vi "StateLimeLight.vi"(0 "Master State":enum16{"Normal", "Climb"}(ring)) -> ()   [LabVIEW 2020]
doc: "This VI manages the LimeLight pipelines and LimeLight targeting LED mode."
uses:
  driverdata.vi
  sensordata.vi
  robotoutputs.vi
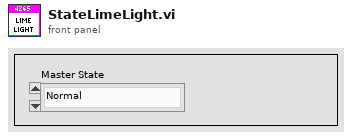
[diagram p1: front panel]
types:
  T1 = enum16{"Robot-Oriented", "Field-Oriented", "Intake"}
  T2 = enum16{"Side-by-Side", "PiP Main", "PiP Secondary"}
  T3 = enum16{"Boot Up", "Camera Override", "HUB Targeting", "CARGO Tracking"}
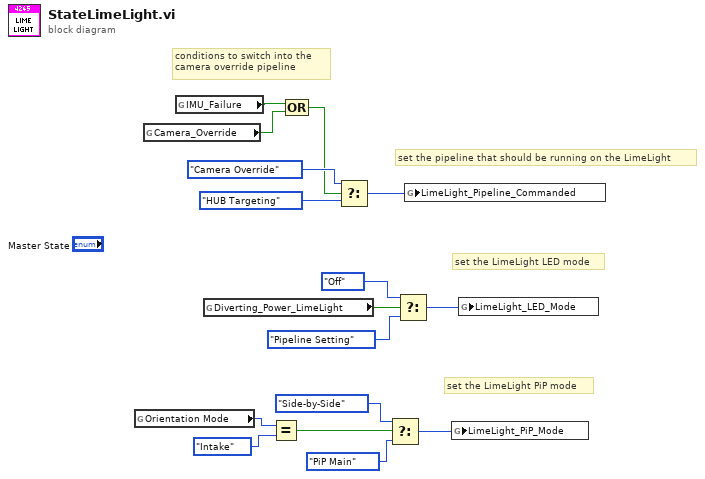
[diagram p0: block diagram]
diagram:
  # "set the LimeLight PiP mode"
  # "set the LimeLight LED mode"
  # "conditions to switch into the \ncamera override pipeline"
  # "set the pipeline that should be running on the LimeLight"
  n1 = global read "robotoutputs.vi" "Orientation Mode"() -> (w3:T1)
  n2 = global read "driverdata.vi" "Camera_Override"() -> (w15:bool)
  n3 = global read "sensordata.vi" "IMU_Failure"() -> (w16:bool)
  n4 = global read "robotoutputs.vi" "Diverting_Power_LimeLight"() -> (w8:bool)
  n5 = Equal?(x=w3, y=T1."Intake") -> (x = y?=w1:bool)
  n6 = Compound Arithmetic op=OR(w16, w15) -> (w13:bool)
  n7 = Select(t=T3."Camera Override", s=w13, f=T3."HUB Targeting") -> (s? t:f=w7:T3)
  n8 = Select(t=T2."Side-by-Side", s=w1, f=T2."PiP Main" ("LimeLight_PiP_Mode")) -> (s? t:f=w6:T2)
  n9 = Select(t=enum16{"Pipeline Setting", "Off", "Blink", "On"}."Off", s=w8, f=enum16{"Pipeline Setting", "Off", "Blink", "On"}."Pipeline Setting") -> (s? t:f=w9:enum16{"Pipeline Setting", "Off", "Blink", "On"})
  n10 = global write "robotoutputs.vi" "LimeLight_Pipeline_Commanded"(w7) -> ()
  n11 = global write "robotoutputs.vi" "LimeLight_PiP_Mode"(w6) -> ()
  n12 = global write "robotoutputs.vi" "LimeLight_LED_Mode"(w9) -> ()
